vi "CreateClass.vi"(7 "PythonConverter_BD in":refnum<class "PyConvBD.lvclass">, 8 "error in":errorcluster, 11 "CaseStructure in":refnum<class "CaseStructure.lvclass">) -> (0 "error out":errorcluster, 3 "CaseStructure out":refnum<class "CaseStructure.lvclass">, 4 "class":string, 5 "PythonConverter_BD out":refnum<class "PyConvBD.lvclass">)   [LabVIEW 2014, in "Raspberry Pi Compatible Compiler for LabVIEW.lvlib" / "CaseStructure.lvclass"]
uses:
  CaseStructure.lvclass
  Python/PythonConverter_BD/PyConvBD.lvclass
  Structure/Structure.lvclass/Structure.ctl
  Diagram/Diagram.lvclass
  Python/Parsing/Python Functions.lvlib
  Structure/Structure.lvclass
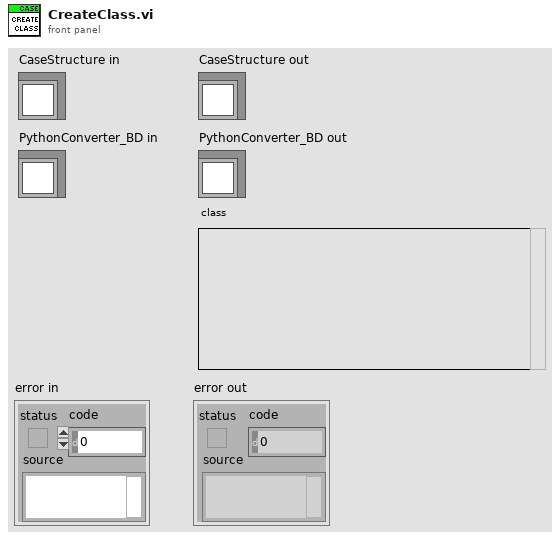
[diagram p1: front panel]
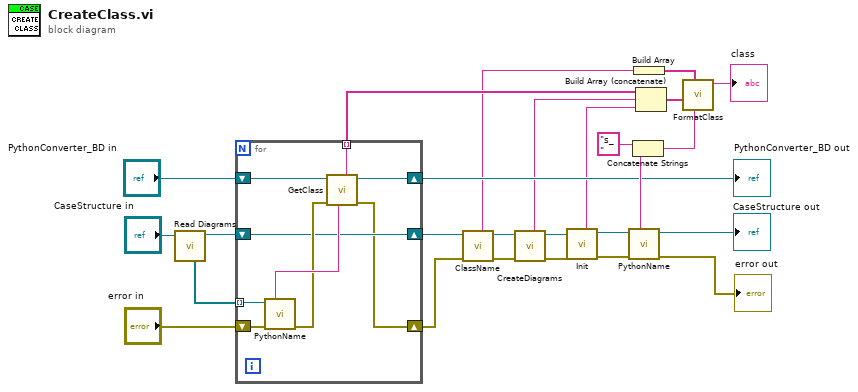
[diagram p0: block diagram]
diagram:
  n1 = call "Read Diagrams.vi"("Structure in"="CaseStructure in") -> ("Structure out"=w20:refnum<class "CaseStructure.lvclass">, "Diagrams"=w22:refnum<class "Diagram.lvclass">[])  [unwired: 7 in]
  n2 = for {
    tunnel: w22 -> [w35] mode=indexing
    shift-right: [w30] -> w19
    shift-left: "PythonConverter_BD in" -> [w34]
    shift-right: [w31] -> w6
    shift-left: w20 -> [w31]
    tunnel: [w29] -> w15 mode=indexing
    shift-right: [w27] -> w4
    shift-left: "error in" -> [w28]
    n3 = call-dynamic "PythonName.vi"("error in"=w28, "Diagram in"=w35) -> ("error out"=w32:errorcluster, "UID"=w33:string)  [unwired: 6 in, 2 out]
    n4 = call "GetClass.vi"("name"=w33, "error in"=w32, "PythonConverter_BD in"=w34) -> ("error out"=w27:errorcluster, "PythonConverter_BD out"=w30:refnum<class "PyConvBD.lvclass">, "class"=w29:string)  [unwired: 4 in]
  }
  "PythonConverter_BD out" <- w19
  n5 = call "ClassName.vi"("error in"=w4, "CaseStructure in"=w6) -> ("error out"=w3:errorcluster, "CaseStructure out"=w5:refnum<class "CaseStructure.lvclass">, "class name"=w2:string)  [unwired: 5 in]
  n6 = call-dynamic "CreateDiagrams.vi"("error in"=w3, "Structure in"=w5) -> ("error out"=w10:errorcluster, "Structure out"=w11:refnum<class "CaseStructure.lvclass">, "create_diagrams"=w14:string)  [unwired: 5 in]
  n7 = call-dynamic "Init.vi"("error in"=w10, "CaseStructure in"=w11) -> ("error out"=w8:errorcluster, "CaseStructure out"=w9:refnum<class "CaseStructure.lvclass">, "__init__"=w7:string)  [unwired: 5 in]
  n8 = call-dynamic "PythonName.vi"("error in"=w8, "Node in"=w9) -> ("error out"=→"error out":errorcluster, "Node out"=→"CaseStructure out":refnum<class "CaseStructure.lvclass">, "UID"=w25:string)  [unwired: 6 in, 1 out]
  n9 = Concatenate Strings("s_" ("format string"), w25) -> (w24:string)
  n10 = Build Array(w2) -> (w1:string[])
  n11 = Build Array (concatenate)(w15, w14, w7) -> (w13:string[])
  n12 = call "FormatClass.vi"("name"=w24, "parameters/ancestors"=w1, "body"=w13) -> ("python"=→"class":string)  [unwired: 8 in]
